vi "Handle Mouse Down.vi"(6 "Button":u16, 8 "error in (no error)":errorcluster, 9 "Double Click":bool, 10 "Coords":T1, 11 "DataGrid in":refnum<class "DataGrid.lvclass">) -> (0 "error out":errorcluster, 2 "Discard?":bool, 3 "DataGrid out":refnum<class "DataGrid.lvclass">)   [LabVIEW 2017, in "DataGrid.lvclass"]
uses:
  DataGrid.lvclass
  <vilib>/Utility/miscctls.llb/LVPoint32TypeDef.ctl
  Write Current Edit Position.vi
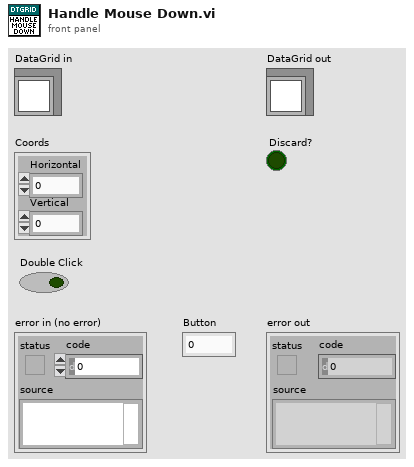
[diagram p1: front panel]
types:
  T1 = typedef "LVPoint32TypeDef.ctl" = cluster{"Horizontal":i32, "Vertical":i32}
  T2 = typedef "LVRowAndColumnTypeDef.ctl" = cluster{"Row":i32, "Column":i32}
  T3 = typedef "Mouse Down Action.ctl" = enum16{"Do Nothing", "Sort Column", "Edit Only", "Add Row and Edit"}
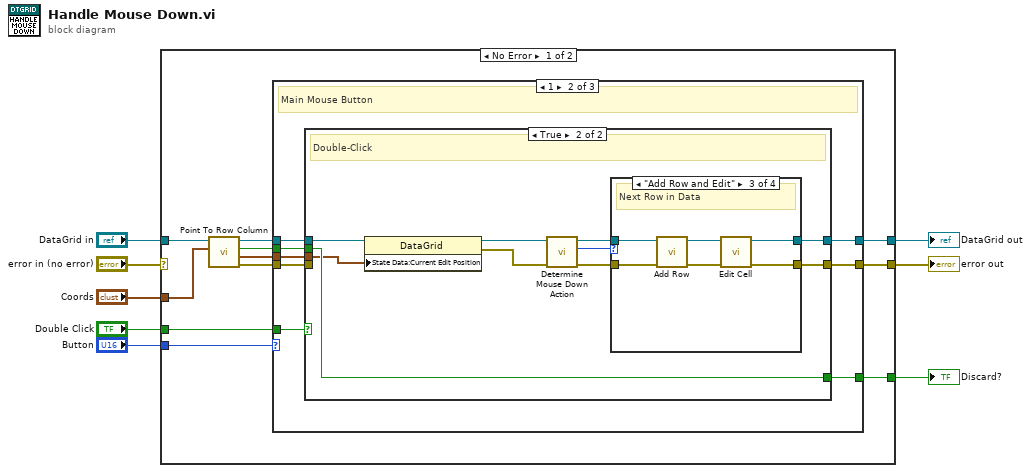
[diagram p0: block diagram]
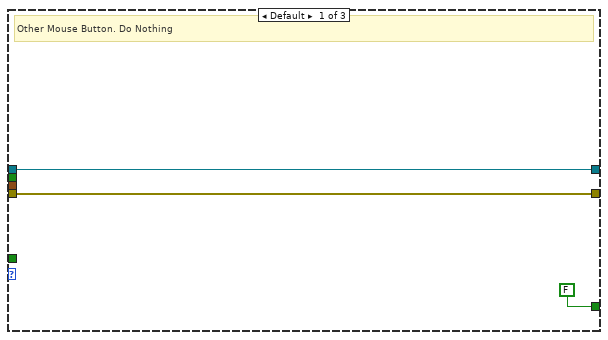
[diagram p2: hidden frame]
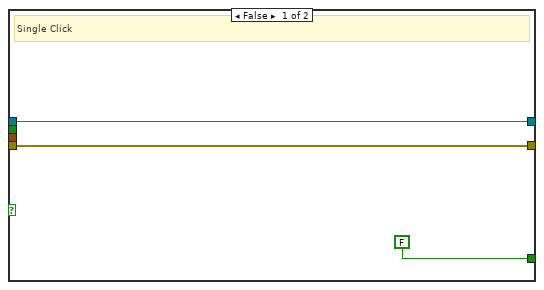
[diagram p3: hidden frame]
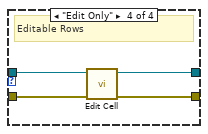
[diagram p6: hidden frame]
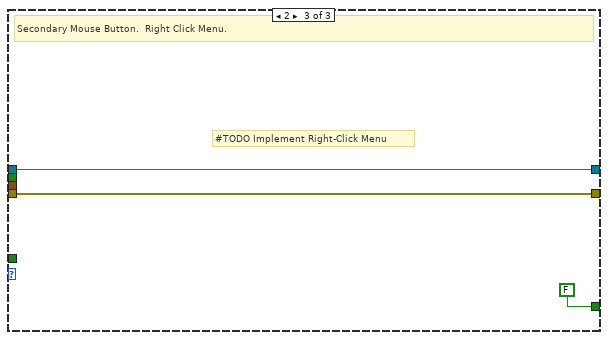
[diagram p7: hidden frame]
diagram:
  n1 = case shown="No Error" "error in (no error)" {
    selector: "error in (no error)" -> [_ w62]
    tunnel: [w16 w62] -> w7
    tunnel: [w15 w61] -> w5
    tunnel: "DataGrid in" -> [w19 w61]
    tunnel: "Coords" -> [w18 _]
    tunnel: "Double Click" -> [w12 _]
    tunnel: [w10 _] -> w3
    tunnel: "Button" -> [w9 _]
    frame No Error {
      n2 = call-dynamic "Point To Row Column.vi"("Point"=w18, "MulticolumnListbox in"=w19) -> ("error out"=w17:errorcluster, "Cell Position"=w14:T2, "In Bounds?"=w11:bool, "MulticolumnListbox out"=w13:refnum<class "DataGrid.lvclass">)  [unwired: 5 in, 1 out]
      n3 = case shown="1" w9 {
        tunnel: w17 -> [w21 w30 w59]
        tunnel: [w21 w29 w59] -> w16
        tunnel: [w22 w28 w60] -> w15
        tunnel: w14 -> [_ w27 _]
        tunnel: w13 -> [w22 w26 w60]
        tunnel: w12 -> [_ w25 _]
        tunnel: w11 -> [_ w24 _]
        tunnel: [FALSE ("In Bounds?") w23 FALSE ("In Bounds?")] -> w10
        frame Default {
          # "Other Mouse Button. Do Nothing"
        }
        frame 1 {
          # "Main Mouse Button"
          n4 = case shown="True" w25 {
            tunnel: w30 -> [w32 _]
            tunnel: [w32 w43] -> w29
            tunnel: [w33 w42] -> w28
            tunnel: w27 -> [_ w34]
            tunnel: w26 -> [w33 w37]
            tunnel: w24 -> [_ w38]
            tunnel: [FALSE w38] -> w23
            frame False {
              # "Single Click"
            }
            frame True {
              # "Double-Click"
              n5 = property class="DataGrid"(reference=w37, "State Data:Current Edit Position"=w34) -> (reference out=w36:refnum<class "DataGrid.lvclass">, error out=w35:errorcluster)  [unwired: 1 in]
              n6 = call "Determine Mouse Down Action.vi"("error in (no error)"=w35, "DataGrid in"=w36) -> ("error out"=w41:errorcluster, "Action"=w39:T3, "DataGrid out"=w40:refnum<class "DataGrid.lvclass">)  [unwired: 7 in]
              n7 = case shown="\"Add Row and Edit\"" w39 {
                tunnel: w41 -> [w44 w46 w50 w54]
                tunnel: [w44 w46 w53 w57] -> w43
                tunnel: [w45 w47 w52 w56] -> w42
                tunnel: w40 -> [w45 w47 w51 w55]
                frame "Do Nothing" {
                  # "Beyond data.  Do nothing."
                }
                frame "Sort Column" {
                  # "#TODO Implement Sort"
                  # "Sort Column"
                }
                frame "Add Row and Edit" {
                  # "Next Row in Data"
                  n8 = call "Add Row.vi"("error in (no error)"=w50, "DataGrid in"=w51) -> ("error out"=w48:errorcluster, "DataGrid out"=w49:refnum<class "DataGrid.lvclass">)  [unwired: 8 in]
                  n9 = call "Edit Cell.vi"("error in (no error)"=w48, "DataGrid in"=w49) -> ("error out"=w53:errorcluster, "DataGrid out"=w52:refnum<class "DataGrid.lvclass">)  [unwired: 8 in]
                }
                frame "Edit Only" {
                  # "Editable Rows"
                  n10 = call "Edit Cell.vi"("error in (no error)"=w54, "DataGrid in"=w55) -> ("error out"=w57:errorcluster, "DataGrid out"=w56:refnum<class "DataGrid.lvclass">)  [unwired: 8 in]
                }
              }
            }
          }
        }
        frame 2 {
          # "#TODO Implement Right-Click Menu"
          # "Secondary Mouse Button.  Right Click Menu."
        }
      }
    }
    frame Error {
    }
  }
  "error out" <- w7
  "DataGrid out" <- w5
  "Discard?" <- w3
